vi "Kelvinox_set_excitation.vi"(6 "Temperature":dbl, 7 "LS_Excitation old":dbl) -> (2 "Change of Excitation?":bool, 3 "LS_Excitation new":dbl)   [LabVIEW 2019]
uses:
  Instrument_Setup.vi
panel:
  out "Path":path
  out "Excitation parameter":string(combo)
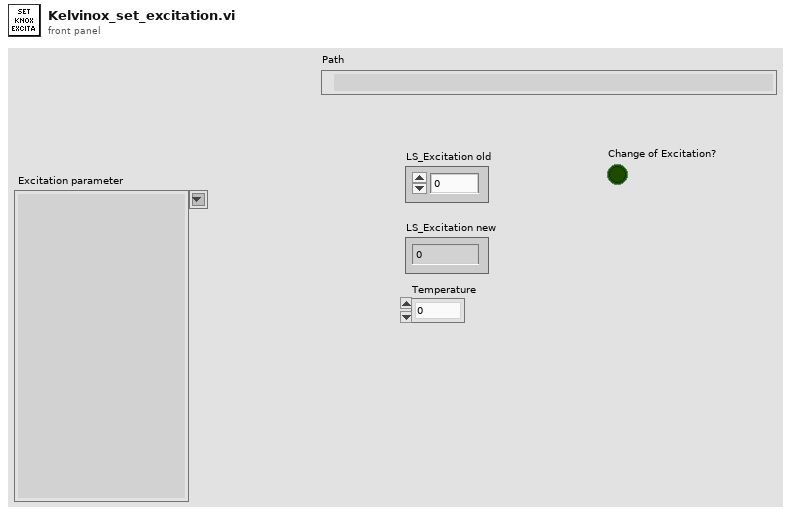
[diagram p1: front panel]
types:
  T1 = enum16{"open", "replace", "create", "open or create", "replace or create", "replace or create with confirmation"}
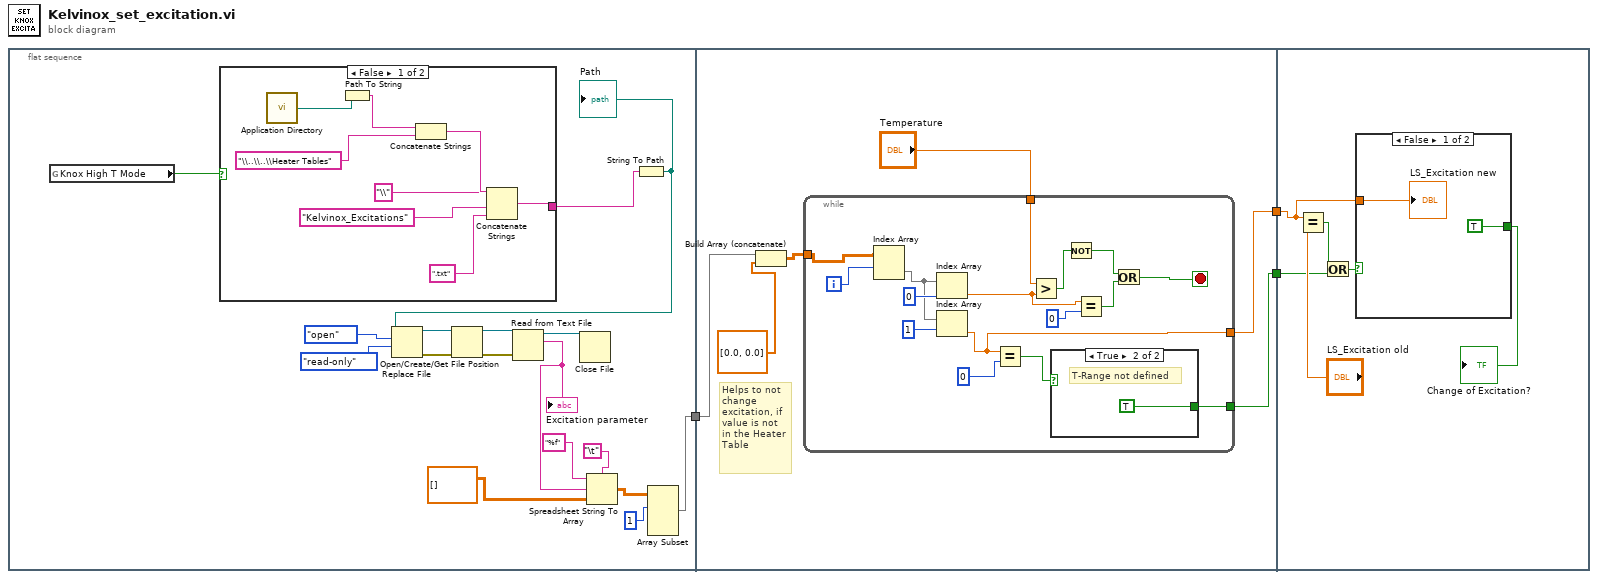
[diagram p0: block diagram]
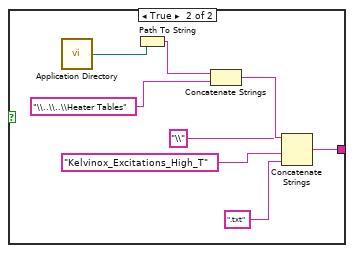
[diagram p2: hidden frame]
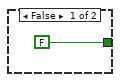
[diagram p3: hidden frame]
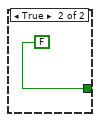
[diagram p4: hidden frame]
diagram:
  n1 = flat-sequence {
    tunnel: [w7] -> w3
    tunnel: w3 -> [w39]
    tunnel: [w42] -> w2
    tunnel: [w40] -> w1
    tunnel: w2 -> [w65]
    tunnel: w1 -> [w61]
    frame #0 {
      n2 = global read "Instrument_Setup.vi" "Knox High T Mode"() -> (w5:bool)
      n3 = case shown="False" w5 {
        tunnel: [w21 w29] -> w4
        frame False {
          n4 = call <vilib>:"Application Directory.vi"() -> ("Application Directory"=w28:path)
          n5 = Path To String(path=w28) -> (string=w27:string)
          n6 = Concatenate Strings(w27, "\\..\\..\\Heater Tables") -> (w25:string)
          n7 = Concatenate Strings(w25, "\\", "Kelvinox_Excitations", ".txt") -> (w21:string)
        }
        frame True {
          n8 = call <vilib>:"Application Directory.vi"() -> ("Application Directory"=w36:path)
          n9 = Path To String(path=w36) -> (string=w35:string)
          n10 = Concatenate Strings(w35, "\\..\\..\\Heater Tables") -> (w33:string)
          n11 = Concatenate Strings(w33, "\\", "Kelvinox_Excitations_High_T", ".txt") -> (w29:string)
        }
      }
      n12 = String To Path(string=w4) -> (path=w13:path)
      "Path" <- w13
      n13 = Open/Create/Replace File(file path (use dialog)=w13, operation (0:open)=T1."open", access (0:read/write)=enum16{"read/write", "read-only", "write-only"}."read-only") -> (refnum out=w18:refnum<file>, error out=w17:errorcluster)  [unwired: 3 in, 1 out]
      n14 = Get File Position(4:w17, 7:w18) -> (0:w15:errorcluster, 3:w16:refnum<file>)  [unwired: 1 out]
      n15 = Read from Text File(file (use dialog)=w16, error in=w15) -> (refnum out=w14:refnum<file>, text=w12:string)  [unwired: 2 in, 2 out]
      "Excitation parameter" <- w12
      n16 = Close File(refnum=w14) -> ()  [unwired: 1 in, 2 out]
      n17 = Spreadsheet String To Array(delimiter (Tab)="\t", format string="%f", spreadsheet string=w12, array type (2D Dbl)=dbl[][] []) -> (array=w8:dbl[][])
      n18 = Array Subset(array=w8, index (row)=1) -> (w7:dbl[][])  [unwired: 3 in]
    }
    frame #1 {
      # "Helps to not\nchange\nexcitation, if\nvalue is not\nin the Heater\nTable"
      n19 = Build Array (concatenate)(w39, dbl[] [0.0, 0.0]) -> (w38:dbl[][])
      n20 = while {
        tunnel: w38 -> [w58]
        tunnel: [w45] -> w42
        tunnel: "Temperature" -> [w54]
        tunnel: [w44] -> w40
        i -> [w43]
        stop <- w48 stop-if-true
        n21 = Index Array(array=w58, index (row)=w43) -> (element=w55:dbl[])  [unwired: 1 in]
        n22 = Index Array(array=w55, index=0) -> (element=w50:dbl)
        n23 = Index Array(array=w55, index=1) -> (element=w45:dbl)
        n24 = Equal?(x=w45, y=0) -> (x = y?=w46:bool)
        n25 = Greater?(x=w54, y=w50) -> (0:w53:bool)
        n26 = case shown="True" w46 {
          tunnel: [FALSE TRUE] -> w44
          frame False {
          }
          frame True {
            # "T-Range not defined"
          }
        }
        n27 = Not(x=w53) -> (.not. x?=w52:bool)
        n28 = Equal?(x=w50, y=0) -> (x = y?=w51:bool)
        n29 = Or(x=w52, y=w51) -> (x .or. y?=w48:bool)
      }
    }
    frame #2 {
      n30 = Equal?(x=w65, y="LS_Excitation old") -> (x = y?=w63:bool)
      n31 = Or(x=w63, y=w61) -> (x .or. y?=w62:bool)
      n32 = case shown="False" w62 {
        tunnel: w65 -> [w68 _]
        tunnel: [TRUE FALSE] -> w64
        frame False {
          "LS_Excitation new" <- w68
        }
        frame True {
        }
      }
      "Change of Excitation?" <- w64
    }
  }
